vi "Auto_Initialization.vi"   [LabVIEW 2014]
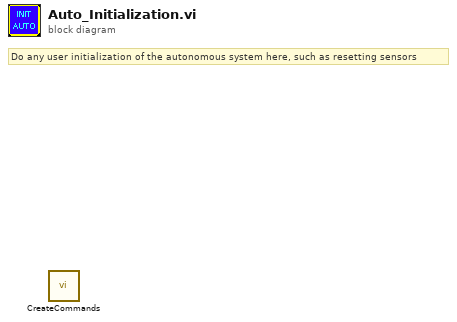
[diagram p0: block diagram]
diagram:
  # "Do any user initialization of the autonomous system here, such as resetting sensors"
  n1 = call "CreateCommands.vi"() -> ()  [unwired: 1 in]
